vi "append default parameters list.vi"(8 "default parameters in":string[](array[string]), 9 "parameter found?":bool, 10 "Key":string, 11 "Section":string) -> (0 "default parameters out":string[](array[string]))   [LabVIEW 2018]
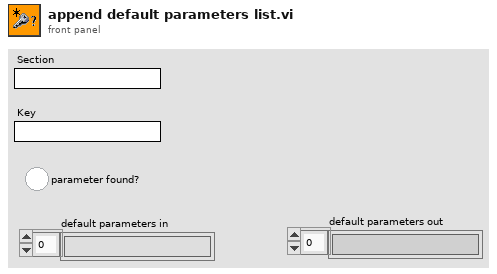
[diagram p1: front panel]
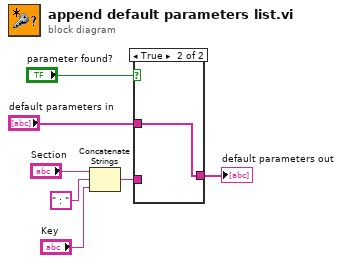
[diagram p0: block diagram]
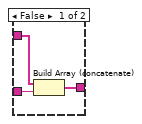
[diagram p2: hidden frame]
diagram:
  n1 = Concatenate Strings("Section", " : " ("string"), "Key") -> (w3:string)
  n2 = case shown="True" "parameter found?" {
    tunnel: "default parameters in" -> [w10 w11]
    tunnel: w3 -> [w9 _]
    tunnel: [w8 w11] -> w2
    frame False {
      n3 = Build Array (concatenate)(w10, w9) -> (w8:string[])
    }
    frame True {
    }
  }
  "default parameters out" <- w2
